vi "Ping Example.vi"() -> ()   [LabVIEW 2012, in "LIFA Ultrasonic Distance.lvlib"]
uses:
  LIFA Ultrasonic Distance.lvlib
  <vilib>/LabVIEW Interface for Arduino/LabVIEW Interface for Arduino.lvlib
  <vilib>/LabVIEW Interface for Arduino/Type Defs/Board Type.ctl
  Get Distance/PING Get Distance.vi
panel:
  out "Distance History (cm)":dbl(graph)
  in  "stop":bool
  # "1.  Upload the provided LIFA firmware.\n\n2.  If using a board other than the Arduino UNO, change the parameters for Init.vi on the block diagram.\n\n3.  Wire the signal pin of the sensor to Arduino pin 8. \n\n4.  Run the VI."
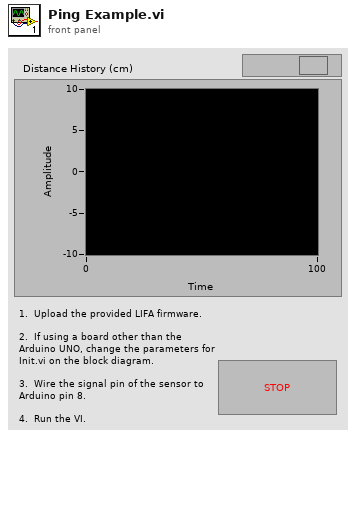
[diagram p1: front panel]
types:
  T1 = typedef "LabVIEW Interface for Arduino.lvlib/Board Type.ctl" = enum16{"Uno", "Dimuelanove w/Atmega 328", "Mega 2560"}
  T2 = typedef "LabVIEW Interface for Arduino.lvlib/Arduino Resource.ctl" = cluster{"VISA resource":refnum<visa-resource-name>, "Board Type":T1, "Connection Type":enum8{"USB / Serial"}, "Bytes Per Packet (15)":u8}
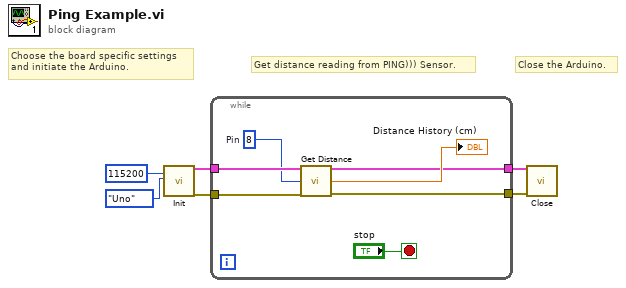
[diagram p0: block diagram]
diagram:
  # "Close the Arduino."
  # "Get distance reading from PING))) Sensor."
  # "Choose the board specific settings\nand initiate the Arduino."
  n1 = call <vilib>:"Init.vi"("Baud Rate (115200)"=u32 115200, "Board Type (Uno)"=Board_Type."Uno") -> ("Arduino Resource"=w6:T2, "error out"=w5:errorcluster)  [unwired: 16 in]
  n2 = while {
    tunnel: w6 -> [w12]
    tunnel: w5 -> [w11]
    tunnel: [w9] -> w3
    tunnel: [w7] -> w4
    stop <- "stop" stop-if-true
    w10 = u8 8  # Pin
    n3 = call-poly "Get Distance.vi"("Arduino Resource"=w12, "Pin"=w10, "error in (no error)"=w11) -> ("Arduino Resource"=w7:T2, "Distance (cm)"=→"Distance History (cm)":dbl, "error out"=w9:errorcluster)  [unwired: 10 in]
  }
  n4 = call <vilib>:"Close.vi"("Arduino Resource"=w4, "error in"=w3) -> ()  [unwired: 13 in, 1 out]
